vi "CTRE_Phoenix_MotorControl_Set.vi"(4 "Demand1":dbl, 6 "DemandType":T1(ring), 8 "error in (no error)":errorcluster, 9 "Output":dbl, 10 "Control Mode":T2 items=["PercentOutput"=0, "Position"=1, "Velocity"=2, "Current"=3, "Follower"=5, "MotionProfile"=6, "MotionMagic"=7, "MotionProfileArc"=10, "Disabled"=15], 11 "PhoenixMotorControlDevRef":T3={"DeviceStatus"={"status"=FALSE, "code"=0, "source"=""}, "Type"=enum."PWM", "PWM"={"PWM Channel"=enum."PWM 1", "DeadBand"={"Name"="", "maxPositivePwm"=0, "minPositivePwm"=0, "centerPwm"=0, "maxNegativePwm"=0, "minNegativePwm"=0, "angularRange"=0}}, "CAN"={"Device Number"=0, "SetOutput VI Ref"=variant(enum8{"Percent VBus", "Current", "Speed", "Position", "Voltage"} enum."Percent VBus"), "GetOutput VI Ref"=variant(refnum<k1> refnum), "Enable VI Ref"=variant(dbl 12.0), "Disable VI Ref"=variant(enum8{"Percent VBus", "Speed", "Position", "Slave", "Unchanged / Invalid", "Voltage Compensation", "Current", "Motion Profile"} enum."Percent VBus"), "Data"=variant}, "Invert"=FALSE, "DIO PWM"={"PWM \"Enable\" Channel"=enum."Invalid", "DIOChannel"=enum."Invalid", "PWM Rate"=0.0}}) -> (0 "error out":errorcluster, 3 "PhoenixMotorControlDevRef":T3={"DeviceStatus"={"status"=FALSE, "code"=0, "source"=""}, "Type"=enum."PWM", "PWM"={"PWM Channel"=enum."PWM 1", "DeadBand"={"Name"="", "maxPositivePwm"=0, "minPositivePwm"=0, "centerPwm"=0, "maxNegativePwm"=0, "minNegativePwm"=0, "angularRange"=0}}, "CAN"={"Device Number"=0, "SetOutput VI Ref"=variant(enum8{"Percent VBus", "Current", "Speed", "Position", "Voltage"} enum."Percent VBus"), "GetOutput VI Ref"=variant(refnum<k1> refnum), "Enable VI Ref"=variant(dbl 12.0), "Disable VI Ref"=variant(enum8{"Percent VBus", "Speed", "Position", "Slave", "Unchanged / Invalid", "Voltage Compensation", "Current", "Motion Profile"} enum."Percent VBus"), "Data"=variant}, "Invert"=FALSE, "DIO PWM"={"PWM \"Enable\" Channel"=enum."Invalid", "DIOChannel"=enum."Invalid", "PWM Rate"=0.0}})   [LabVIEW 2018]
doc: "Sets the Output and Control Mode of the Motor Controller.\n\n<b>Control Mode</b> Sets the appropriate output on the talon, depending on the mode.\n<b>Output</b> The output value to apply\n<b>DemandType</b> The demand type for demand1.\n Neutral: Ignore demand1 and apply no change to output.\n AuxPID: Use demand 1 to set the target for auxiliary PID 1.\n ArbitraryFeedForward: Use demand1 as an arbitrary additive value to the demand 0 output\n<b>Demand1</b> Supplemental output value. Units match the set mode."
uses:
  <vilib>/Rock Robotics/WPI/MotorControl/WPI_MotorControlDeviceRef.ctl
  <vilib>/Rock Robotics/WPI/MotorControl/WPI_MotorControlType.ctl
  <vilib>/Rock Robotics/SystemInterfaces/DIO/FPGA_DIOPWMChannel.ctl
  <vilib>/Rock Robotics/WPI/PWM/WPI_PWMDeadband.ctl
  <vilib>/Rock Robotics/SystemInterfaces/DIO/FPGA_DIOChannel.ctl
  Controls/CTRE_Phoenix_MotorControl_ControlMode.ctl
  Controls/CTRE_Phoenix_MotorControl_DevRefData.ctl
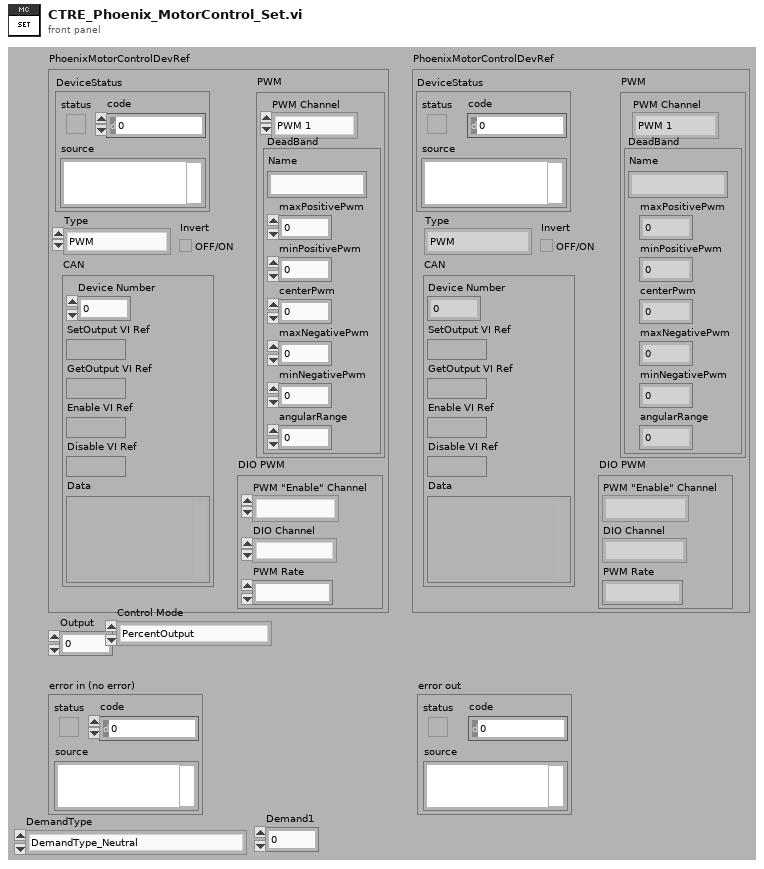
[diagram p1: front panel]
types:
  T1 = enum16{"DemandType_Neutral", "DemandType_AuxPID", "DemandType_ArbitraryFeedForward"}
  T2 = typedef "CTRE_Phoenix_MotorControl_ControlMode.ctl" = u16
  T3 = typedef "WPI_MotorControlDeviceRef.ctl" = cluster{"DeviceStatus":errorcluster, "Type":T4, "PWM":cluster{"PWM Channel":T5, "DeadBand":T6}, "CAN":cluster{"Device Number":u8, "SetOutput VI Ref":variant, "GetOutput VI Ref":variant, "Enable VI Ref":variant, "Disable VI Ref":variant, "Data":variant}, "Invert":bool, "DIO PWM":cluster{"PWM \"Enable\" Channel":T5, "DIOChannel":T7, "PWM Rate":dbl}}
  T4 = typedef "WPI_MotorControlType.ctl" = enum16{"PWM", "CAN", "DIO PWM"}
  T5 = typedef "FPGA_DIOPWMChannel.ctl" = enum8{"PWM 0", "PWM 1", "PWM 2", "PWM 3", "PWM 4", "PWM 5", "PWM 6", "PWM 7", "PWM 8", "PWM 9", "PWM MXP 0", "PWM MXP 1", "PWM MXP 2", "PWM MXP 3", "PWM MXP 4", "PWM MXP 5", "PWM MXP 6", "PWM MXP 7", "PWM MXP 8", "PWM MXP 9", "Invalid"}
  T6 = typedef "WPI_PWMDeadband.ctl" = cluster{"Name":string, "maxPositivePwm":i32, "minPositivePwm":i32, "centerPwm":i32, "maxNegativePwm":i32, "minNegativePwm":i32, "angularRange":u16}
  T7 = typedef "FPGA_DIOChannel.ctl" = enum8{"DIO 0", "DIO 1", "DIO 2", "DIO 3", "DIO 4", "DIO 5", "DIO 6", "DIO 7", "DIO 8", "DIO 9", "DIO MXP 0", "DIO MXP 1", "DIO MXP 2", "DIO MXP 3", "DIO MXP 4", "DIO MXP 5", "DIO MXP 6", "DIO MXP 7", "DIO MXP 8", "DIO MXP 9", "DIO MXP 10", "DIO MXP 11", "DIO MXP 12", "DIO MXP 13", "DIO MXP 14", "DIO MXP 15", "SPI Port CS1", "SPI Port CS2", "SPI Port CS3", "SPI Port MISO", "SPI Port MOSI", "Invalid"}
  T8 = typedef "CTRE_Phoenix_MotorControl_DevRefData.ctl" = cluster{"Library":path, "handle":u64, "Control Mode":T2, "UsageFrame":u32, "RefNumName":string, "arbID":u32}
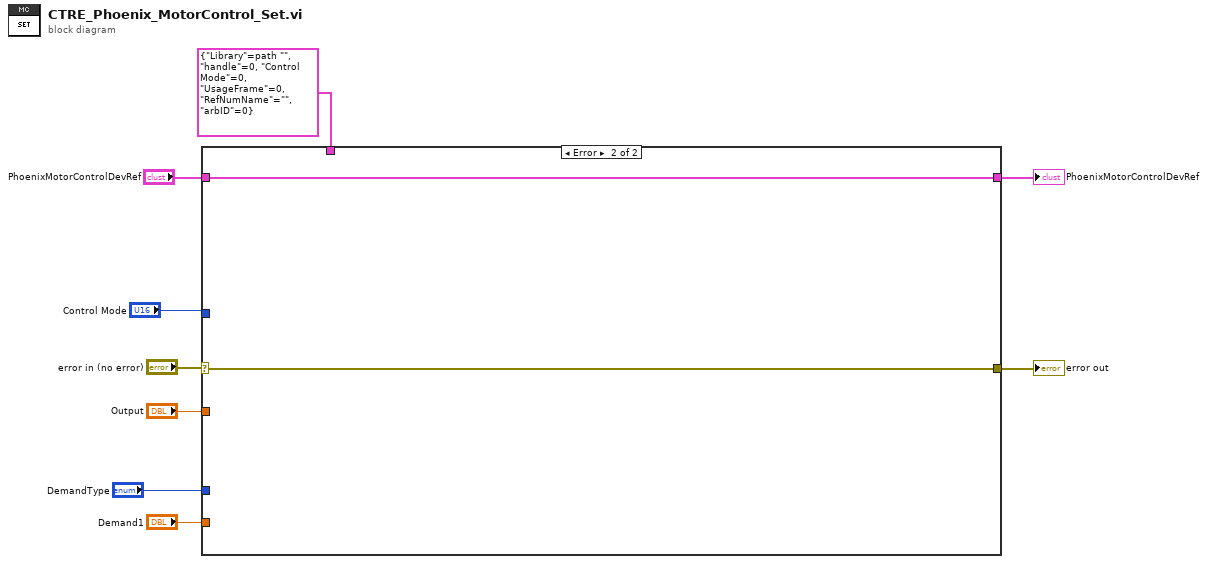
[diagram p0: block diagram]
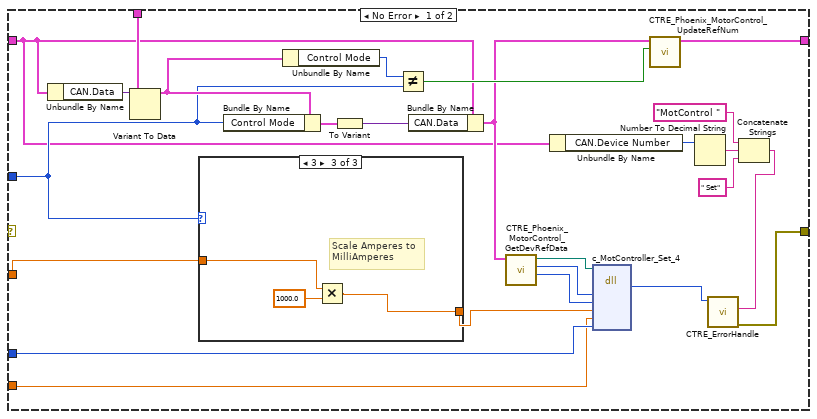
[diagram p2: hidden frame]
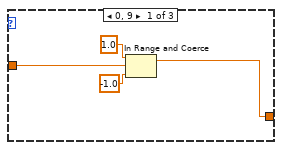
[diagram p3: hidden frame]
diagram:
  n1 = case shown="Error" "error in (no error)" {
    selector: "error in (no error)" -> [_ w44]
    tunnel: [w12 w44] -> w9
    tunnel: [w29 w43] -> w7
    tunnel: "PhoenixMotorControlDevRef" -> [w15 w43]
    tunnel: "Control Mode" -> [w26 _]
    tunnel: "Output" -> [w34 _]
    tunnel: T8 {"Library"=path "", "handle"=0, "Control Mode"=0, "UsageFrame"=0, "RefNumName"="", "arbID"=0} ("Cluster") -> [w33 _]
    tunnel: "DemandType" -> [w11 _]
    tunnel: "Demand1" -> [w10 _]
    frame No Error {
      n2 = Unbundle By Name(w15) -> ("CAN.Data"=w30:variant)
      n3 = Variant To Data(type=w33, Variant=w30) -> (data=w28:T8)  [unwired: 1 in, 1 out]
      n4 = case shown="3" w26 {
        tunnel: [w35 w39 w40] -> w20
        tunnel: w34 -> [w36 w39 w42]
        frame 0, 9 {
          n5 = In Range and Coerce(upper limit=1.0, x=w36, lower limit=-1.0) -> (coerced(x)=w35:dbl)  [unwired: 1 out]
        }
        frame 5, Default {
        }
        frame 3 {
          # "Scale Amperes to\nMilliAmperes"
          n6 = Multiply(x=w42, y=1000.0) -> (x*y=w40:dbl)
        }
      }
      n7 = Bundle By Name(cluster=w28, "Control Mode"=w26) -> (w31:T8)
      n8 = Unbundle By Name(w28) -> ("Control Mode"=w27:T2)
      n9 = To Variant(anything=w31) -> (Variant=w32:variant)
      n10 = Not Equal?(x=w27, y=w26) -> (x != y?=w25:bool)
      n11 = Bundle By Name(cluster=w15, "CAN.Data"=w32) -> (w24:T3)
      n12 = call "CTRE_Phoenix_MotorControl_GetDevRefData.vi"("PhoenixMotorControlDevRef"=w24) -> ("Talon SRX Mode"=w21:T2, "handle"=w22:u64, "Library"=w23:path)  [unwired: 4 in, 4 out]
      n13 = Unbundle By Name(w15) -> ("CAN.Device Number"=w19:u8)
      n14 = dll-call lib="?" fn="c_MotController_Set_4"(path in=w23, "handle"=w22, "mode"=w21, "demand0"=w20, "demand1"=w10, "demand1Type"=w11) -> ("return type"=w13:i32)  [unwired: 7 in, 2 out]
      n15 = call "CTRE_Phoenix_MotorControl_UpdateRefNum.vi"("Update"=w25, "PhoenixMotorControlDevRef"=w24) -> ("PhoenixMotorControlDevRef"=w29:T3)  [unwired: 9 in]
      n16 = Number To Decimal String(number=w19) -> (decimal integer string=w18:string)  [unwired: 1 in]
      n17 = Concatenate Strings("MotControl " ("string"), w18, " Set" ("string")) -> (w14:string)
      n18 = call "CTRE_ErrorHandle.vi"("origin"=w14, "code"=w13) -> ("error out"=w12:errorcluster)  [unwired: 9 in]
    }
    frame Error {
    }
  }
  "PhoenixMotorControlDevRef" <- w7
  "error out" <- w9
